vi "Get Maximum Exposure.vi"(8 "error in (no error)":errorcluster, 11 "MaxExp":sgl) -> (0 "error out":errorcluster, 2 "function return":u32, 3 "MaxExp out":sgl)   [LabVIEW 2014, in "atmcd32d.lvlib"]
doc: "unsigned int WINAPI GetMaximumExposure(float * MaxExp);"
uses:
  atmcd32d.lvlib
  atmcd32d.dll
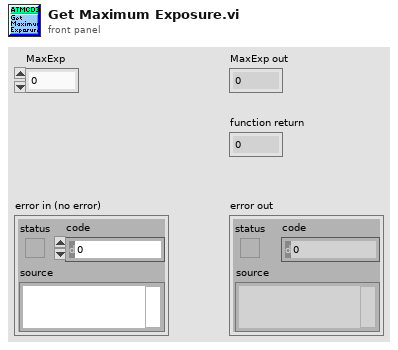
[diagram p1: front panel]
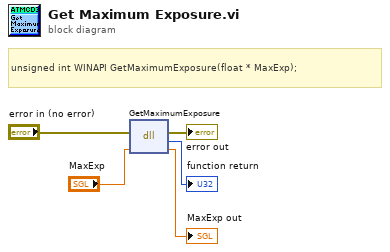
[diagram p0: block diagram]
diagram:
  # "unsigned int WINAPI GetMaximumExposure(float * MaxExp);"
  n1 = dll-call lib="C:/Users/Bakir/Documents/Lambda2-Testing/lib/Andorlib/atmcd32d.*" fn="GetMaximumExposure"(error in="error in (no error)", "MaxExp"="MaxExp") -> (error out=→"error out":errorcluster, →"function return":u32, "MaxExp"=→"MaxExp out":sgl)  [unwired: 2 in, 1 out]
